vi "conv_taille_vers_n.vi"(0 "taille":string) -> (1 "val_effectif":i32, 2 "ch_effectif":string)   [LabVIEW 2010, in "lv_04.lvlib"]
uses:
  lv_04.lvlib
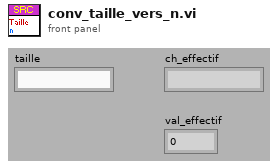
[diagram p1: front panel]
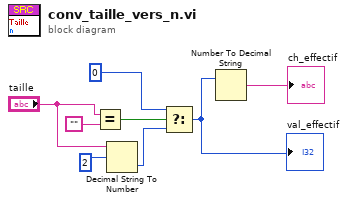
[diagram p0: block diagram]
diagram:
  n1 = Equal?(x="taille", y="") -> (x = y?=w3:bool)
  n2 = Decimal String To Number(string="taille", offset=2 ("offset (0)")) -> (number=w7:i32)  [unwired: 1 in, 1 out]
  n3 = Select(t=0, s=w3, f=w7) -> (s? t:f=w8:i32)
  "val_effectif" <- w8
  n4 = Number To Decimal String(number=w8) -> (decimal integer string=→"ch_effectif":string)  [unwired: 1 in]
